vi "loadDataNodeBegin.vi"(8 "error in (no error)":errorcluster, 10 "XML Refnum in":refnum<file>, 11 "Channel_FXP in":refnum<class "Channel_FXP.lvclass">) -> (0 "error out":errorcluster, 2 "XML Refnum out":refnum<file>, 3 "Channel_FXP out":refnum<class "Channel_FXP.lvclass">)   [LabVIEW 2013, in "Channel_FXP.lvclass"]
doc: "Part of the file loading process. Occurs at the beginning of a node being loaded. Loads the common xceDataNode data name and description."
uses:
  Channel_FXP.lvclass
  Channel/Channel.lvclass
  XML Parser/XML Parser.lvclass
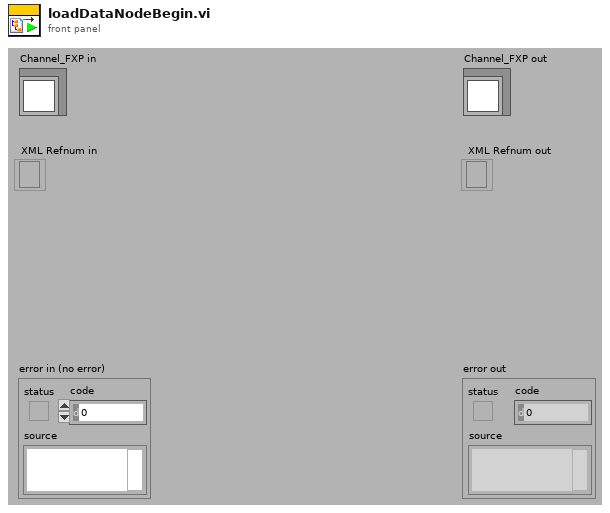
[diagram p1: front panel]
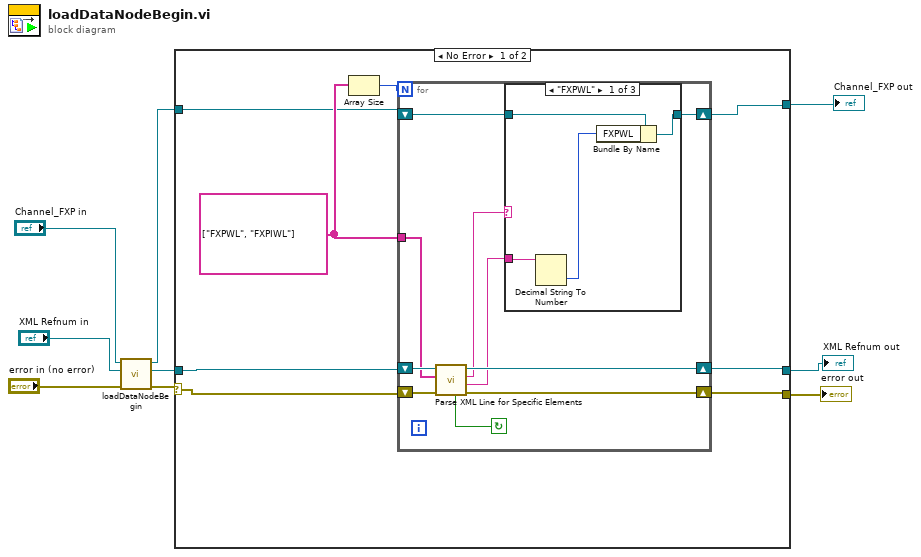
[diagram p0: block diagram]
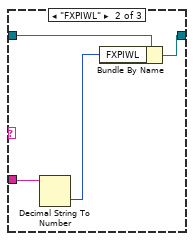
[diagram p2: hidden frame]
diagram:
  n1 = call-parent "loadDataNodeBegin.vi"("error in (no error)"="error in (no error)", "XML Refnum in"="XML Refnum in", "Channel in"="Channel_FXP in") -> ("error out"=w6:errorcluster, "XML Refnum out"=w5:refnum<file>, "Channel out"=w2:refnum<class "Channel_FXP.lvclass">)  [unwired: 6 in]
  n2 = case shown="No Error" w6 {
    selector: w6 -> [w13 w38]
    tunnel: w5 -> [w14 w39]
    tunnel: [w11 w39] -> w3
    tunnel: [w10 w38] -> w4
    tunnel: w2 -> [w15 w37]
    tunnel: [w12 w37] -> w1
    frame No Error {
      w17 = string[] ["FXPWL", "FXPIWL"] ("Token List")
      n3 = Array Size(array=w17) -> (size(s)=w16:i32)
      n4 = for {
        N: w16 -> [_]
        shift-right: [w25] -> w11
        shift-left: w14 -> [w27]
        shift-right: [w24] -> w10
        shift-left: w13 -> [w26]
        shift-right: [w18] -> w12
        shift-left: w15 -> [w19]
        tunnel: w17 -> [w23]
        stop <- w22 continue-if-true
        n5 = call "Parse XML Line for Specific Elements.vi"("error in (no error)"=w26, "Elements"=w23, "XML Refnum in"=w27) -> ("error out"=w24:errorcluster, "Value"=w20:string, "Element Name"=w21:string, "XML Refnum out"=w25:refnum<file>, "Element Found"=w22:bool)  [unwired: 4 in]
        n6 = case shown="\"FXPWL\"" w21 {
          tunnel: w20 -> [w29 w33 _]
          tunnel: w19 -> [w31 w35 w36]
          tunnel: [w30 w34 w36] -> w18
          frame "FXPWL" {
            n7 = Decimal String To Number(string=w29) -> (number=w28:i32)  [unwired: 2 in, 1 out]
            n8 = Bundle By Name(cluster=w31, "FXPWL"=w28) -> (w30:refnum<class "Channel_FXP.lvclass">)
          }
          frame "FXPIWL" {
            n9 = Decimal String To Number(string=w33) -> (number=w32:i32)  [unwired: 2 in, 1 out]
            n10 = Bundle By Name(cluster=w35, "FXPIWL"=w32) -> (w34:refnum<class "Channel_FXP.lvclass">)
          }
          frame Default {
          }
        }
      }
    }
    frame Error {
    }
  }
  "error out" <- w4
  "Channel_FXP out" <- w1
  "XML Refnum out" <- w3
